vi "get video encoeding info.vi"(8 "error in":errorcluster, 11 "Path":path) -> (0 "error out":errorcluster, 1 "Valid?":bool, 3 "output 1":timestamp=timestamp(3382438998 s since 1904-01-01))   [LabVIEW 2023, in "File Classes.lvlib" / "Video File.lvclass"]
uses:
  Video File.lvclass
  <vilib>/Utility/error.llb/Trim Whitespace One-Sided.vi
  Video File.lvclass/Video File.ctl
panel:
  out "standard error":string
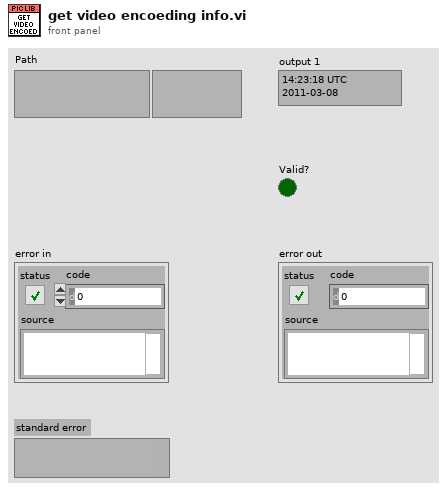
[diagram p1: front panel]
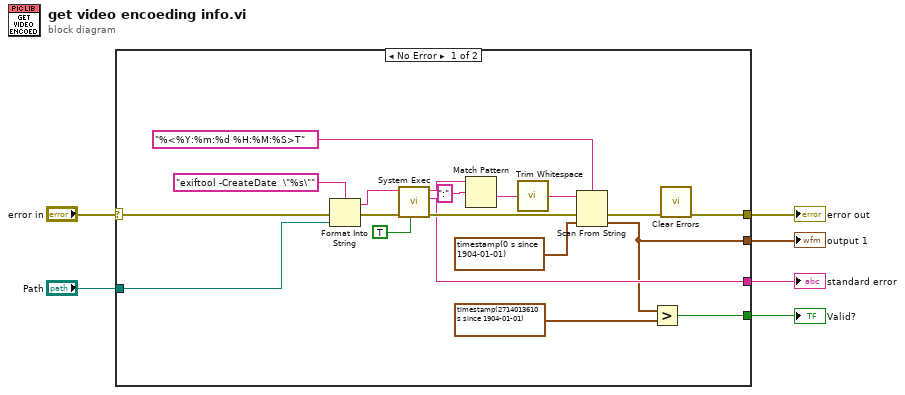
[diagram p0: block diagram]
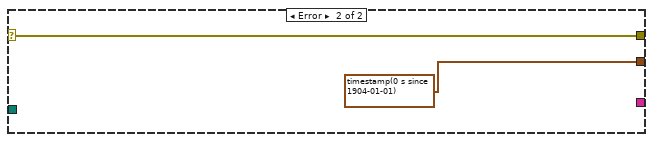
[diagram p2: hidden frame]
diagram:
  n1 = case shown="No Error" "error in" {
    selector: "error in" -> [w13 w27]
    tunnel: [w8 timestamp(0 s since 1904-01-01)] -> w6
    tunnel: "Path" -> [w19 _]
    tunnel: [w10 w27] -> w4
    tunnel: [w12 _] -> w2
    tunnel: [w7 _] -> w1
    frame No Error {
      n2 = Format Into String(format string="exiftool -CreateDate  \"%s\"" ("command line"), error in=w13, w19) -> (resulting string=w17:string, error out=w15:errorcluster)  [unwired: 1 in]
      n3 = call <vilib>:"System Exec.vi"("run minimized? (F)"=TRUE, "error in (no error)"=w15, "command line"=w17) -> ("error out"=w14:errorcluster, "standard error"=w12:string, "standard output"=w24:string)  [unwired: 5 in, 1 out]
      n4 = Match Pattern(string=w24, regular expression=":") -> (after substring=w22:string)  [unwired: 1 in, 3 out]
      n5 = call <vilib>:"Trim Whitespace.vi"("string"=w22) -> ("trimmed string"=w20:string)  [unwired: 1 in]
      n6 = Scan From String(format string="%<%Y:%m:%d %H:%M:%S>T", input string=w20, error in=w14, default 1=timestamp(0 s since 1904-01-01)) -> (error out=w16:errorcluster, output 1=w8:timestamp)  [unwired: 1 in, 2 out]
      n7 = Greater?(x=w8, y=timestamp(2714013610.1 s since 1904-01-01) ("Time Stamp")) -> (0:w7:bool)
      n8 = call <vilib>:"Clear Errors.vi"("error in (no error)"=w16) -> ("error out"=w10:errorcluster)  [unwired: 5 in, 1 out]
    }
    frame Error {
    }
  }
  "output 1" <- w6
  "error out" <- w4
  "standard error" <- w2
  "Valid?" <- w1
